vi "pointListToOverlay.vi"(1 "points":i32[][](array[numeric])) -> (0 "overlay (XYZ)":cluster{"X":i32, "Y":i32, "Z":i32}[](array[cluster]))   [LabVIEW 2017]
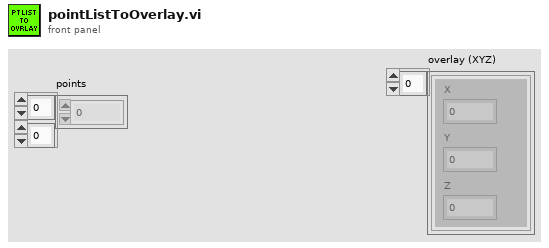
[diagram p1: front panel]
types:
  T1 = cluster{"Numeric":i32, "Numeric":i32, "Numeric":i32}
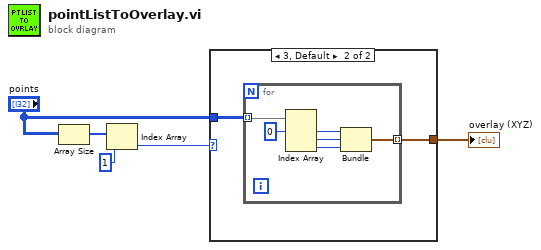
[diagram p0: block diagram]
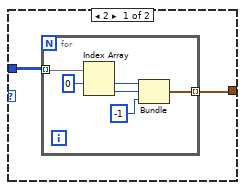
[diagram p2: hidden frame]
diagram:
  n1 = Array Size(array="points") -> (size(s)=w5:i32[])
  n2 = Index Array(array=w5, index=1) -> (element=w1:i32)
  n3 = case shown="3, Default" w1 {
    tunnel: "points" -> [w7 w15]
    tunnel: [w6 w14] -> w2
    frame 2 {
      n4 = for {
        tunnel: w7 -> [w13] mode=indexing
        tunnel: [w9] -> w6 mode=indexing
        n5 = Index Array(array=w13, index #1=0 ("index")) -> (element #1=w11:i32, element #2=w10:i32)  [unwired: 1 in]
        n6 = Bundle("Numeric"=w11, "Numeric"=w10, -1) -> (w9:cluster{"Numeric":i32, "Numeric":i32, i32})  [unwired: 1 in]
      }
    }
    frame 3, Default {
      n7 = for {
        tunnel: w15 -> [w21] mode=indexing
        tunnel: [w16] -> w14 mode=indexing
        n8 = Index Array(array=w21, index #1=0 ("index")) -> (element #1=w19:i32, element #2=w18:i32, element #3=w17:i32)  [unwired: 2 in]
        n9 = Bundle("Numeric"=w19, "Numeric"=w18, "Numeric"=w17) -> (w16:T1)  [unwired: 1 in]
      }
    }
  }
  "overlay (XYZ)" <- w2
